vi "multiline_string_test.vi"() -> ()   [LabVIEW 2014]
panel:
  in  "Stop Button":bool
  out "output string":string
  in  "String":string
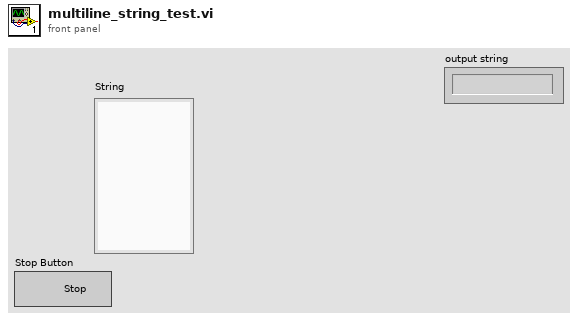
[diagram p1: front panel]
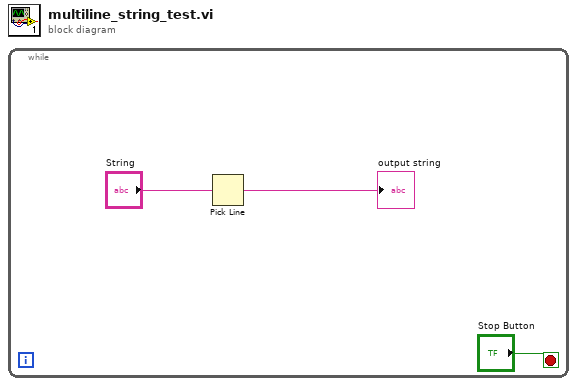
[diagram p0: block diagram]
diagram:
  n1 = while {
    stop <- "Stop Button" stop-if-true
    n2 = Pick Line(multi-line string="String") -> (output string=→"output string":string)  [unwired: 2 in]
  }
